vi "S-Vector.vi"(10 "i-th word":i32, 11 "Round":i32) -> (2 "s":i32)   [LabVIEW 2013, in "MD5.lvlib" / "MD5.lvclass"]
uses:
  MD5.lvclass
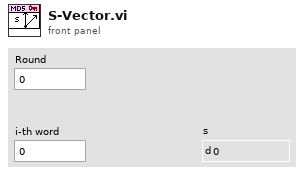
[diagram p1: front panel]
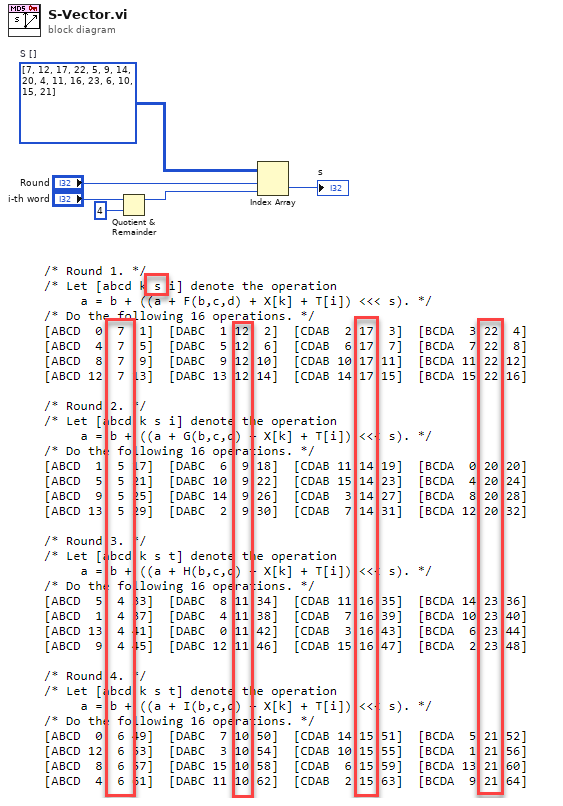
[diagram p0: block diagram]
diagram:
  w5 = i32[][] [[7, 12, 17, 22], [5, 9, 14, 20], [4, 11, 16, 23], [6, 10, 15, 21]]  # S []
  n1 = Quotient & Remainder(x="i-th word", y=4) -> (x-y*floor(x/y)=w1:i32)  [unwired: 1 out]
  n2 = Index Array(array=w5, index (row)="Round", index (col)=w1) -> (element=→"s":i32)
